vi "JudgePowerEnergy.vi"(4 "error out 2":errorcluster caption="error In", 6 "通道":enum16{"Channel 1", "Channel 2"}(ring), 7 "connection In":refnum<k5>) -> (0 "error out":errorcluster, 1 "是否可以测能量":bool, 2 "是否可以测功率":bool, 3 "connection ID":refnum<k5>)   [LabVIEW 2018]
panel:
  out "数字":u32
  out "添加的数组":string[](array[string])
  out "数据输出 2":string
  out "数据输出":string
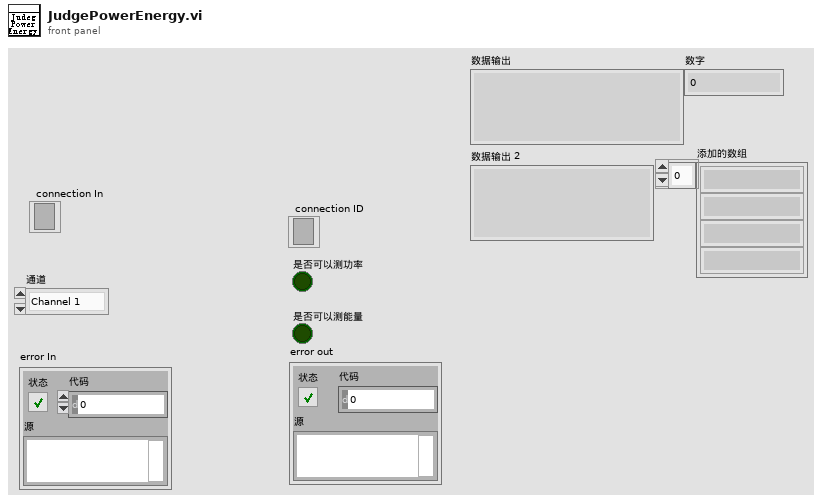
[diagram p1: front panel]
types:
  T1 = enum16{"Standard", "Buffered", "CRLF", "Immediate"}
  T2 = typedef "IMAQ Image.ctl" = refnum<image>
  T3 = cluster{"示波器":cluster{"Channel (0:Channel 1)":enum16{"Channel 1", "Channel 2", "Channel 3", "Channel 4"}, "电压范围":dbl, "触发电压":dbl, "时间范围":dbl, " 示波器VISA":refnum<visa-resource-name>, "时间范围 标签":u64, "电压范围 标签":u64, "触发电压 标签":u64, "输入阻抗/Ω":u64}, "光谱仪":cluster{"SpecDataReference":refnum<queue>, "grating center":dbl, "Exposure Time (s)":dbl, "是否进行详细设置":bool, " 开始通信检查":bool, "通信成功？":bool, "波长":dbl}, " 近场相机":cluster{"曝光时间/us":dbl, "模拟增益":i32, "控制套接字":i32, "IP 地址":string, " 采集套接字":i32, "  版本号":i32, "ImageData":T2, "  增益最大":i32, "  增益最小":i32, " 曝光最大":i32, " 曝光最小":i32, " 帧速":i32, " 同步切换":i32, "  曝光缩放":i32, "Camera Source":refnum<k21>, "近场X范围":dbl, "近场Y范围":dbl, "单个像元大小/um":dbl, "相机距离原点位置":dbl[], "是否测量发散角":bool, "光束类型(发散T)":bool, "聚焦透镜焦距mm":dbl}, " 偏振仪":cluster{"电压范围":u64, "触发电压":u64, "时间范围":u64, "波长范围":enum16{"可见光 400-700nm", "近红外 700-1100nm"}, "可见光偏振测量仪VISA":refnum<visa-resource-name>, "近红外偏振测量仪VISA":refnum<visa-resource-name>}, " 功率计":cluster{"通道":enum16{"Channel 1", "Channel 2"}, "工作波长":u32, "单位":u64, "时间范围":u64, "IP地址":string, "端口":u32, "是否需要散射片":bool}, "能量计":cluster{"通道":enum16{"Channel 1", "Channel 2"}, "工作波长":u32, "单位":u64, "时间范围":u64, "IP地址":string, "端口":u32, "能量计量程":enum16{"200uJ", "20uJ", "2uJ", "200nJ"}}, "电机":cluster{"Channel (0:Channel 1)":enum16{"Channel 1", "Channel 2", "Channel 3", "Channel 4"}, "电压范围":u64, "触发电压":u64, "时间范围":u64}, " 远场相机":cluster{"曝光时间":i32, "模拟增益":i32, "控制套接字":i32, "IP 地址":string, " 采集套接字":i32, "  版本号":i32, "ImageData":T2, "  增益最大":i32, "  增益最小":i32, " 曝光最大":i32, " 曝光最小":i32, " 帧速":i32, " 同步切换":i32, "  曝光缩放":i32, "ImageData B":T2, "是否远场测量":bool}}
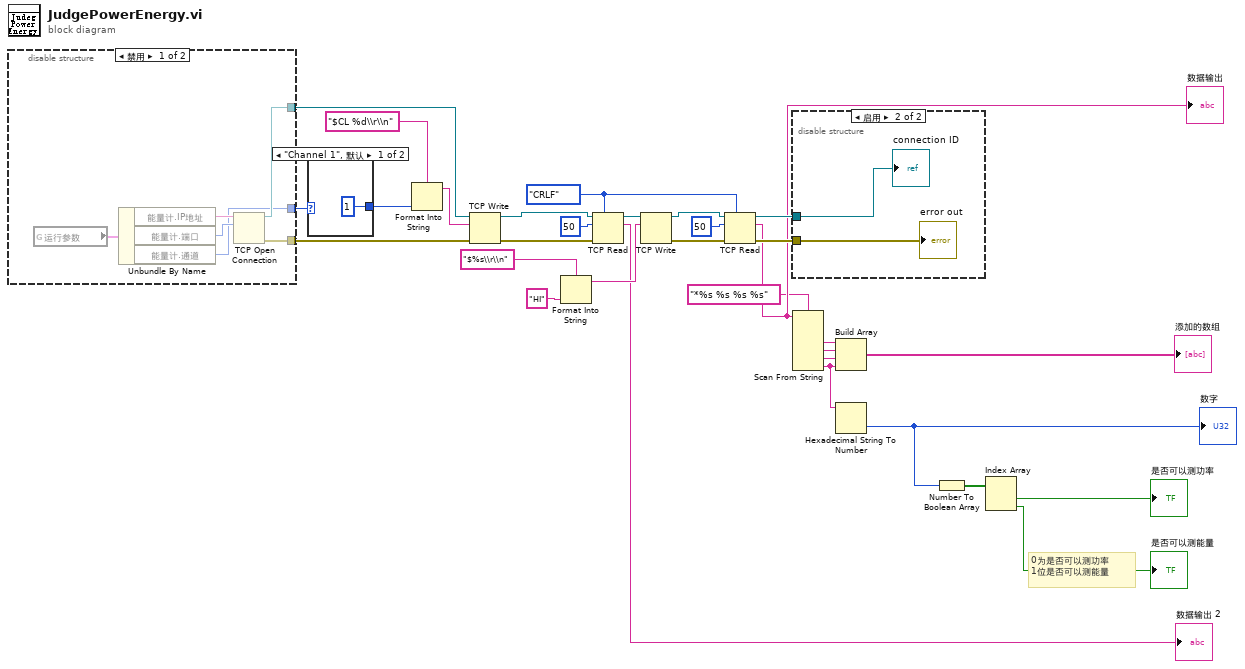
[diagram p0: block diagram]
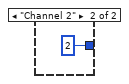
[diagram p2: hidden frame]
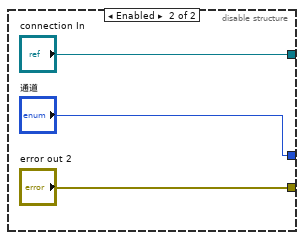
[diagram p3: hidden frame]
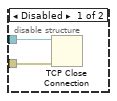
[diagram p4: hidden frame]
diagram:
  w18 = T1."CRLF" ("模式（标准）")
  # "0为是否可以测功率\n1位是否可以测能量"
  n1 = disable-structure shown="禁用" {
    disable-tunnel: [w34 "connection In"] -> w21
    disable-tunnel: [w33 "error out 2"] -> w3
    disable-tunnel: [w32 "通道"] -> w2
    frame Disabled {
      n2 = global read "参数.vi" "运行参数"() -> (w37:T3)
      n3 = Unbundle By Name(w37) -> ("能量计.IP地址"=w36:string, "能量计.端口"=w35:u32, "能量计.通道"=w32:enum16{"Channel 1", "Channel 2"})
      n4 = TCP Open Connection(address=w36, remote port or service name=w35) -> (connection ID=w34:refnum<k5>, error out=w33:errorcluster)  [unwired: 3 in]
    }
    frame Enabled {
    }
  }
  n5 = case shown="\"Channel 1\", 默认" w2 {
    tunnel: [1 ("读取的字节") 2 ("读取的字节")] -> w1
    frame "Channel 1", Default {
    }
    frame "Channel 2" {
    }
  }
  n6 = Format Into String(format string="$CL %d\\r\\n" ("格式字符串"), w1) -> (resulting string=w22:string)  [unwired: 2 in, 1 out]
  n7 = TCP Write(connection ID=w21, data in=w22, error in (no error)=w3) -> (connection ID out=w20:refnum<k5>, error out=w19:errorcluster)  [unwired: 1 in, 1 out]
  n8 = Format Into String(format string="$%s\\r\\n" ("格式字符串"), "HI" ("数据输入")) -> (resulting string=w29:string)  [unwired: 2 in, 1 out]
  n9 = TCP Read(connection ID=w20, bytes to read=50 ("读取的字节"), error in (no error)=w19, 7:w18) -> (connection ID out=w15:refnum<k5>, data out=→"数据输出 2":string)  [unwired: 1 in, 1 out]
  n10 = TCP Write(connection ID=w15, data in=w29) -> (connection ID out=w28:refnum<k5>, error out=w27:errorcluster)  [unwired: 2 in, 1 out]
  n11 = TCP Read(connection ID=w28, bytes to read=50 ("读取的字节"), error in (no error)=w27, 7:w18) -> (connection ID out=w25:refnum<k5>, data out=w14:string, error out=w24:errorcluster)  [unwired: 1 in]
  "数据输出" <- w14
  n12 = disable-structure shown="启用" {
    disable-tunnel: w25 -> [w44 w46]
    disable-tunnel: w24 -> [w43 w45]
    frame Disabled {
      n13 = TCP Close Connection(connection ID=w44, error in (no error)=w43) -> ()  [unwired: 1 in, 2 out]
    }
    frame Enabled {
      "connection ID" <- w46
      "error out" <- w45
    }
  }
  n14 = Scan From String(format string="*%s %s %s %s" ("格式字符串"), input string=w14) -> (output 1=w12:string, output 2=w11:string, output 3=w10:string, output 4=w8:string)  [unwired: 6 in, 3 out]
  n15 = Build Array(w12, w11, w10, w8) -> (→"添加的数组":string[])
  n16 = Hexadecimal String To Number(string=w8) -> (number=w7:u32)  [unwired: 2 in, 1 out]
  "数字" <- w7
  n17 = Number To Boolean Array(number=w7) -> (Boolean array=w6:bool[])
  n18 = Index Array(array=w6) -> (element #1=→"是否可以测功率":bool, element #2=→"是否可以测能量":bool)  [unwired: 2 in]
